vi "ExpectedDepsCheckResults.vi"(0 "ResultsArray":T1[](array[typedef]), 5 "Library Name":string, 7 "Expected Direct Dependencies":string[](array[string]), 9 "Expected Indirect Dependencies":string[](array[string]), 11 "Actual Direct Dependencies":string[](array[string]), 12 "Actual Indirect Dependencies":string[](array[string])) -> (4 "ResultsArray out":T1[](array[typedef]))   [LabVIEW 2019, in "Hawkeye.lvlib"]
uses:
  Hawkeye.lvlib
  Typedefs/DepsCheckResult.ctl
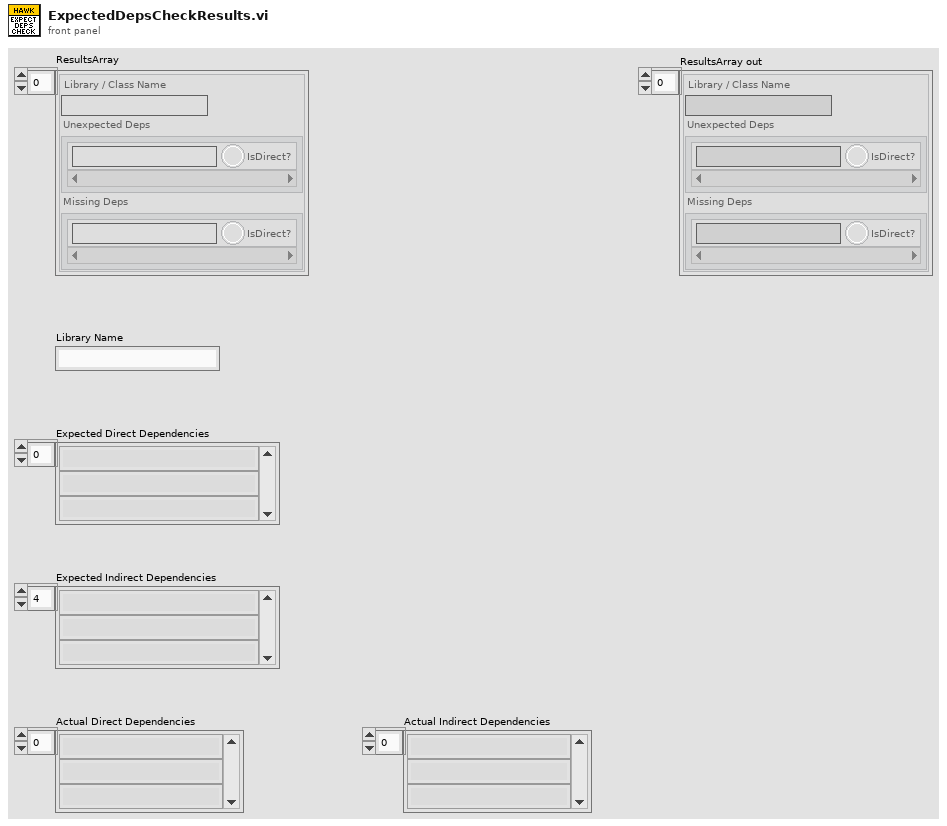
[diagram p1: front panel]
types:
  T1 = typedef "Hawkeye.lvlib/DepsCheckResult.ctl" = cluster{"Library / Class Name":string, "Unexpected Deps":cluster{"Dependency":string, "IsDirect?":bool}[], "Missing Deps":cluster{"Dependency":string, "IsDirect?":bool}[]}
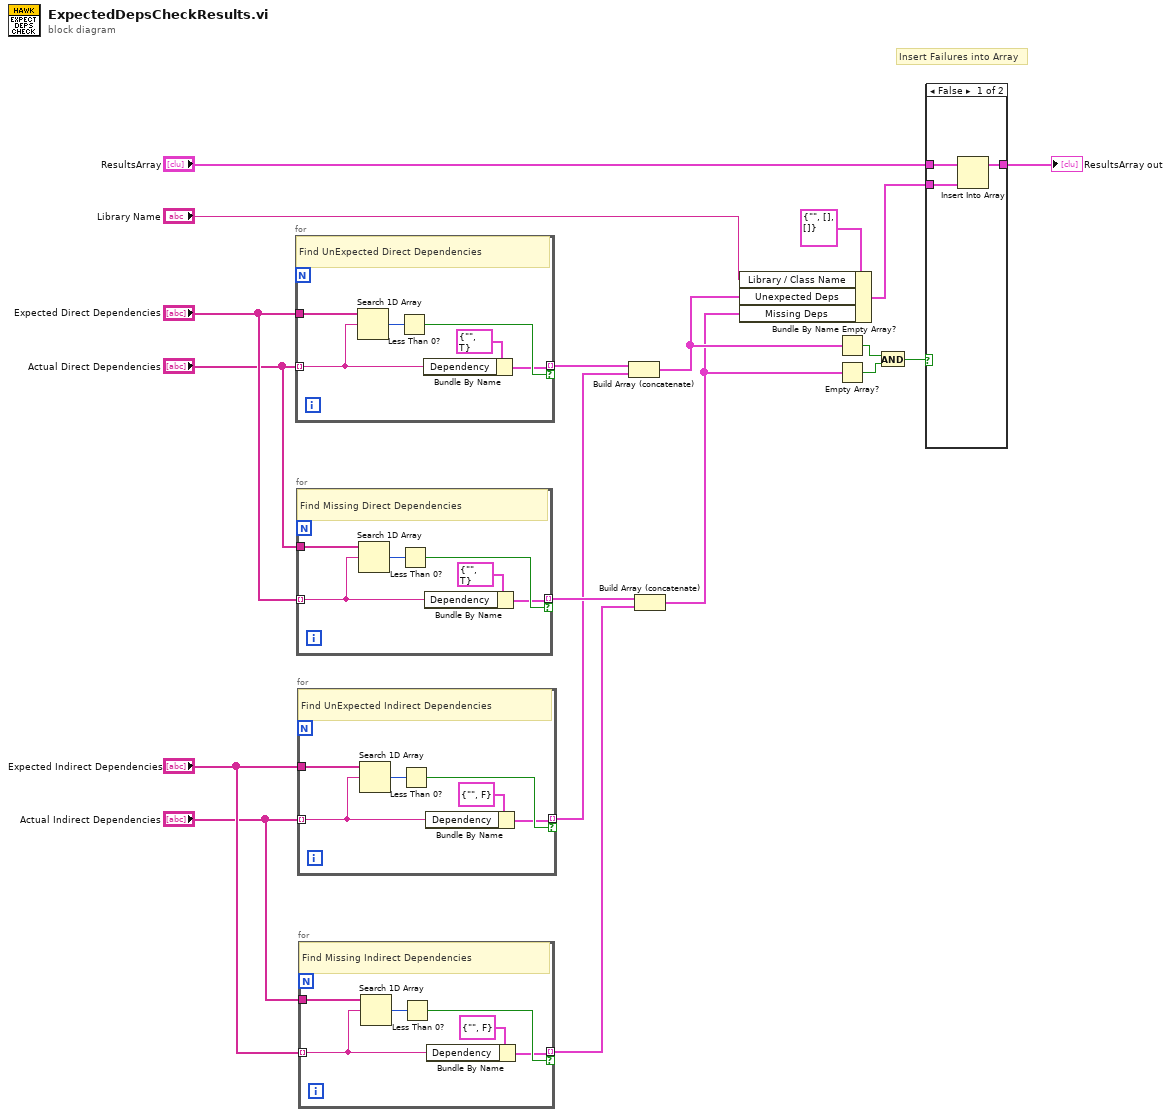
[diagram p0: block diagram]
diagram:
  # "Insert Failures into Array"
  n1 = for {
    tunnel: "Expected Direct Dependencies" -> [w24]
    tunnel: "Actual Direct Dependencies" -> [w19] mode=indexing
    tunnel: [w20] -> w11 mode=indexing if=w22
    # "Find UnExpected Direct Dependencies"
    n2 = Search 1D Array(1D array=w24, element=w19) -> (index of element=w23:i32)  [unwired: 1 in]
    n3 = Less Than 0?(x=w23) -> (x < 0?=w22:bool)
    n4 = Bundle By Name(cluster=cluster{"Dependency":string, "IsDirect?":bool} {"Dependency"="", "IsDirect?"=TRUE} ("Cluster 2"), "Dependency"=w19) -> (w20:cluster{"Dependency":string, "IsDirect?":bool})
  }
  n5 = for {
    tunnel: "Actual Direct Dependencies" -> [w30]
    tunnel: "Expected Direct Dependencies" -> [w25] mode=indexing
    tunnel: [w26] -> w10 mode=indexing if=w28
    # "Find Missing Direct Dependencies"
    n6 = Search 1D Array(1D array=w30, element=w25) -> (index of element=w29:i32)  [unwired: 1 in]
    n7 = Less Than 0?(x=w29) -> (x < 0?=w28:bool)
    n8 = Bundle By Name(cluster=cluster{"Dependency":string, "IsDirect?":bool} {"Dependency"="", "IsDirect?"=TRUE} ("Cluster 2"), "Dependency"=w25) -> (w26:cluster{"Dependency":string, "IsDirect?":bool})
  }
  n9 = for {
    tunnel: "Expected Indirect Dependencies" -> [w36]
    tunnel: "Actual Indirect Dependencies" -> [w31] mode=indexing
    tunnel: [w32] -> w2 mode=indexing if=w34
    # "Find UnExpected Indirect Dependencies"
    n10 = Search 1D Array(1D array=w36, element=w31) -> (index of element=w35:i32)  [unwired: 1 in]
    n11 = Less Than 0?(x=w35) -> (x < 0?=w34:bool)
    n12 = Bundle By Name(cluster=cluster{"Dependency":string, "IsDirect?":bool} {"Dependency"="", "IsDirect?"=FALSE} ("Cluster 2"), "Dependency"=w31) -> (w32:cluster{"Dependency":string, "IsDirect?":bool})
  }
  n13 = for {
    tunnel: "Actual Indirect Dependencies" -> [w42]
    tunnel: "Expected Indirect Dependencies" -> [w37] mode=indexing
    tunnel: [w38] -> w1 mode=indexing if=w40
    # "Find Missing Indirect Dependencies"
    n14 = Search 1D Array(1D array=w42, element=w37) -> (index of element=w41:i32)  [unwired: 1 in]
    n15 = Less Than 0?(x=w41) -> (x < 0?=w40:bool)
    n16 = Bundle By Name(cluster=cluster{"Dependency":string, "IsDirect?":bool} {"Dependency"="", "IsDirect?"=FALSE} ("Cluster 2"), "Dependency"=w37) -> (w38:cluster{"Dependency":string, "IsDirect?":bool})
  }
  n17 = Build Array (concatenate)(w11, w2) -> (w4:cluster{"Dependency":string, "IsDirect?":bool}[])
  n18 = Build Array (concatenate)(w10, w1) -> (w3:cluster{"Dependency":string, "IsDirect?":bool}[])
  n19 = Bundle By Name(cluster=T1 {"Library / Class Name"="", "Unexpected Deps"=[], "Missing Deps"=[]}, "Library / Class Name"="Library Name", "Unexpected Deps"=w4, "Missing Deps"=w3) -> (w13:T1)
  n20 = Empty Array?(array=w4) -> (empty?=w9:bool)
  n21 = Empty Array?(array=w3) -> (empty?=w8:bool)
  n22 = And(x=w9, y=w8) -> (x .and. y?=w7:bool)
  n23 = case shown="False" w7 {
    tunnel: "ResultsArray" -> [w45 w46]
    tunnel: w13 -> [w44 _]
    tunnel: [w43 w46] -> w12
    frame False {
      n24 = Insert Into Array(array=w45, new element=w44) -> (w43:T1[])  [unwired: 1 in]
    }
    frame True {
    }
  }
  "ResultsArray out" <- w12
